vi "Create JSONLFormatter.vi"(8 "error in":errorcluster, 10 "Datetime format":string="%.;%Y-%m-%d %H:%M:%S%3u") -> (0 "error out":errorcluster, 3 "JSONLFormatter out":refnum<class "JSONLFormatter.lvclass">)   [LabVIEW 2016, in "hse-logger.lvlib" / "JSONLFormatter.lvclass"]
doc: "Creates and initializes a new JSONLFormatter object. Optionally specify Datetime format, default is \"%Y-%m-%d %H:%M:%S\"."
uses:
  JSONLFormatter.lvclass
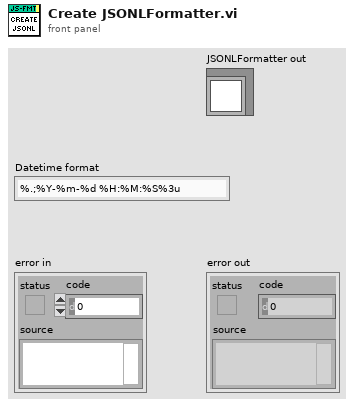
[diagram p1: front panel]
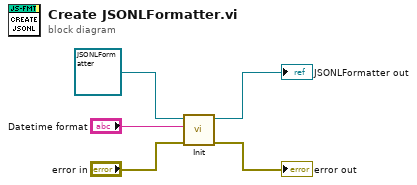
[diagram p0: block diagram]
diagram:
  n1 = call-dynamic "Init.vi"("error in"="error in", "Datetime format"="Datetime format", "Formatter in"=refnum<class "JSONLFormatter.lvclass"> refnum ("JSONLFormatter in")) -> ("error out"=→"error out":errorcluster, "Formatter out"=→"JSONLFormatter out":refnum<class "JSONLFormatter.lvclass">)  [unwired: 7 in]
